vi "Dashboard Main.vi"() -> ()   [LabVIEW 2016]
uses:
  <vilib>/Utility/miscctls.llb/LVRowAndColumnTypeDef.ctl
  <vilib>/event_ctls.llb/eventvkey.ctl
  <vilib>/Rock Robotics/Network Tables/NT Read Numeric Array.vi
  <vilib>/Rock Robotics/WPI/Dashboard/WPI_DashboardLogging Global.vi
panel:
  in  "Camera Settings Right":T1={"Frame Rate"=30, "Compression"=30, "Size"=1, "DB Camera Config"=FALSE} {"Frame Rate" scale=1.0..30.0; "Compression" scale=100.0..-1.0; "Size" items=["640x480", "320x240", "160x120"]}
  in  "Camera Name Right":string(combo)="No Camera Selection"
  out "Camera Info":cluster{"Mbps LED":bool, "Mbps":dbl, "fps":dbl} {"fps" format="%#.1g"; "Mbps" format="%#.1g"}
  in  "Camera Settings":T1={"Frame Rate"=30, "Compression"=30, "Size"=1, "DB Camera Config"=FALSE} {"Frame Rate" scale=1.0..30.0; "Compression" scale=100.0..-1.0; "Size" items=["640x480", "320x240", "160x120"]}
  in  "TCP":refnum<k5>
  in  "Rec Mode":enum32{"Stop", "Record", "Playback"}(radio)
  out "Robot IP":string
  out "Image Message":string="Timeout in Camera Communications"
  in  "Dashboard Tab":T2(tab)
  in  "Select Auto":string(combo)="Select Autonomous ..."
  out "NT Connection":bool
  out "MotorChart R":cluster{"Numeric":dbl, "Numeric":dbl}(graph)
  out "MotorChart L":cluster{"Numeric":dbl, "Numeric":dbl}(graph)
  out "MotorSliders R":cluster{"MotorSlide1":dbl, "MotorSlide2":dbl} {"MotorSlide2" scale=-1.0..1.0 scale format="%#_2e"; "MotorSlide1" scale=-1.0..1.0 scale format="%#_2e"}
  out "MotorSliders L":cluster{"MotorSlide1":dbl, "MotorSlide2":dbl} {"MotorSlide2" scale=-1.0..1.0 scale format="%#_2e"; "MotorSlide1" scale=-1.0..1.0 scale format="%#_2e"}
  out "Gyro":dbl(knob) scale=0.0..360.0
  out "JS1 Z":dbl(slide) scale=-1.0..1.0 scale format="%#_2e"
  out "JS1 Graph":cluster{"X":dbl, "Y":dbl}[](graph)
  out "JS1 Buttons":T3
  out "JS2 Z":dbl(slide) scale=-1.0..1.0 scale format="%#_2e"
  out "JS2 Graph":cluster{"X":dbl, "Y":dbl}[](graph)
  out "JS2 Buttons":T3
  out "Mode":T4(ring)=enum."Auto Disabled"
  out "Camera Image Right":T5(plugin-control)
  in  "DB/String 9":string
  in  "DB/String 8":string
  in  "DB/String 7":string
  in  "DB/String 6":string
  in  "DB/String 5":string
  in  "DB/String 4":string
  in  "DB/String 3":string
  in  "DB/String 2":string
  in  "DB/String 1":string
  in  "DB/String 0":string
  in  "DB/Slider 0":dbl(slide) scale=0.0..5.0
  in  "DB/Slider 1":dbl(slide) scale=0.0..5.0
  in  "DB/Slider 2":dbl(slide) scale=0.0..5.0
  in  "DB/Slider 3":dbl(slide) scale=0.0..5.0
  out "DB/LED 3":bool
  out "DB/LED 2":bool
  out "DB/LED 1":bool
  out "DB/LED 0":bool
  in  "TimedDrive":bool
  in  "DriveTowardTower":bool caption="Tower Drive"
  in  "ReleaseGear":bool
  in  "GrabGear":bool
  in  "Test Slider":dbl(slide) scale=0.0..100.0 scale format="%#_3g"
  in  "On/Off":bool caption="Solenoid"
  in  "Test Name":u16(ring) items=["Select the test to run..."]
  in  "Test Tree":string(tree)
  in  "Motor":cluster{"Value":dbl, "Enable":bool} {"Value" scale=-1.0..1.0 scale format="%#_3g"}
  out "Progress":T6 {"Test Progress" scale=0.0..100.0}
  in  "Rev/Fwd":cluster{"Forward":bool, "Reverse":bool}
  in  "Test Ring":u16(ring) items=["Monochrome", "Color"]
  out "Cmd Status":string
  in  "Execute Command":bool
  in  "Command Params":string[][](table)
  in  "Command Selection":i32(listbox)
  in  "CheckList":i32(listbox)
  in  "Tree":string(tree)
  out "Camera Image":T5(plugin-control)
  out "Background":bool
  in  "Camera Name":string(combo)="No Camera Selection"
  # "HW"
  # "HW"
  # "Joysticks"
  # "Drive Motors"
  # "Front"
  # "Right"
  # "Left"
  # "Back"
  # "This tab is a great place for autonomous settings and robot-specific values.\nPlace controls and indicators inside this tab and match name to\nDashboard Variables on robot. You can also delete this comment."
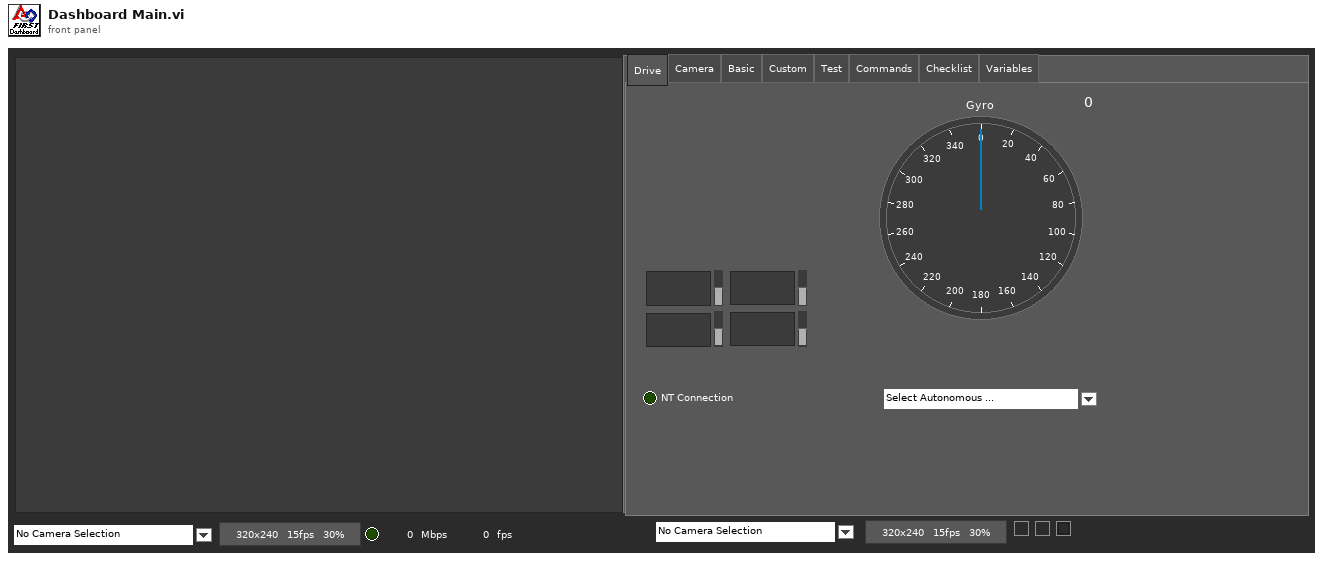
[diagram p1: front panel]
types:
  T1 = cluster{"Frame Rate":i32, "Compression":i32, "Size":u16, "DB Camera Config":bool}
  T2 = enum32{"Drive", "Camera", "Basic", "Custom", "Test", "Commands", "Checklist", "Variables"}
  T3 = cluster{bool, bool, bool, bool, bool, bool, bool, bool, bool, bool, bool, bool}
  T4 = enum8{"Tele-Op Disabled", "Tele-Op Enabled", "Auto Disabled", "Auto Enabled", "Test Disabled", "Test Enabled", "Disconnected", "No Code", "E-Stop"}
  T5 = typedef "IMAQ Image.ctl" = refnum<image>
  T6 = cluster{"Test Progress":u8, "Test Progress Text":string}
  T7 = typedef "Image Type" = u32
  T8 = cluster{"IDs":cluster{"RPC field ID":u16, "Unique ID":u16}, "String":string}
  T9 = enum32{"Drive", "Basic", "Custom", "Test", "Checklist", "Variables"}
  T10 = cluster{"Error Strings":string, "Disable Counts":cluster{u16, u16}, "Rail Faults":cluster{u16, u16, u16}, "Robot IP":string, "DB Mode":u8, "Event Info":cluster{"Name":string, "Type":u8, "Number":u16, "Replay":u8}}
  T11 = cluster{"Storage":cluster{"Disk Free":u64, "RAM Block":u32, "RAM free":u32}, "CPU Utilization":cluster{"CPU % ISR":sgl, "CPU % Time Crit":sgl, "CPU % Timed Str":sgl, "CPU % High":sgl, "CPU % Above":sgl, "CPU % Normal":sgl, "CPU % Low":sgl}, "CAN":cluster{"% Bus Utilization":sgl, "Bus Off Cnt":u32, "TX_FIFO Full Cnt":u32, "Receive Error Cnt":u8, "Transmit Error Cnt":u8}, "HID":cluster{"HID Outputs":u32, "Rumble Low":u16, "Rumble High":u16}[]}
  T12 = cluster{"Status bits":cluster{"Test Mode":bool, "Autonomous":bool, "Enabled":bool, "Code Start":bool, "Brownout":bool, "Reserved 2":bool, "Reserved 3":bool, "E-Stop":bool}, "Code Trace":cluster{"Disabled":bool, "TeleOp":bool, "Auto":bool, "Test":bool}, "Controller Type":enum16{"unknown", "cRIO", "roboRio"}, "Code?":enum16{"unknown", "noCode", "code"}, "Battery V":dbl}
  T13 = cluster{"Control Bits":cluster{"TestMode":bool, "Autonomous":bool, "Enabled":bool, "FMS Present":bool, bool, bool, bool, "E-Stop":bool}, "Team Station ":u8, "Countdown":sgl, "Joystick Values":cluster{"Axes":dbl[], "Buttons":bool[], "POVs":i16[]}[]}
  T14 = cluster{"Axes":dbl[], "Buttons":bool[], "POVs":i16[]}[]
  T15 = cluster{"Axes":dbl[], "Buttons":bool[], "POVs":i16[]}
  T16 = cluster{"Buttons[0]":bool, "Buttons[1]":bool, "Buttons[2]":bool, "Buttons[3]":bool, "Buttons[4]":bool, "Buttons[5]":bool, "Buttons[6]":bool, "Buttons[7]":bool, "Buttons[8]":bool, "Buttons[9]":bool, "Buttons[10]":bool, "Buttons[11]":bool}
  T17 = cluster{"Camera Image":refnum<vi>, "Dashboard Tab":refnum<vi>, "Background":refnum<vi>, "Rec Mode":refnum<vi>, "Test Slider":refnum<vi>, "On/Off ":refnum<vi>, "Test Ring":refnum<vi>, "Rev/Fwd":refnum<vi>, "Test Name":refnum<vi>, "Motor":refnum<vi>, "Progress":refnum<vi>, "CheckList":refnum<vi>, "Tree":refnum<vi>, "Test Tree":refnum<vi>, "Command Params":refnum<vi>, "Command Selection":refnum<vi>, "Execute Command":refnum<vi>, "Cmd Status":refnum<vi>, "Camera Settings":refnum<vi>, "Camera Name":refnum<vi>, "Camera Info":refnum<vi>, "Camera Settings Right":refnum<vi>, "Camera Name Right":refnum<vi>, "Camera Image Right":refnum<vi>}
  T18 = cluster{"Operation":enum16{"Update", "Clear"}, "Color Box":u32}[]
  T19 = typedef "eventvkey.ctl" = enum16{"ASCII", "Enter", "Return", "Shift", "Ctrl", "Alt", "Cmd", "Opt", "Caps", "NumLock", "Clear", "Break", "Up", "Down", "Left", "Right", "Insert", "Delete", "Home", "End", "PageUp", "PageDown", "Escape", "Help", "Pause", "ScrollLock", "F1", "F2", "F3", "F4", "F5", "F6", "F7", "F8", "F9", "F10", "F11", "F12", "F13", "F14", "F15", "F16", "F17", "F18", "F19", "F20", "F21", "F22", "F23", "F24", "Play", "VolumeUp", "VolumeDown", "Mute", "Two Byte Char"}
  T20 = cluster{"Image Size":bool, "Image Type":bool, "Pixel Value":bool, "ROI Information":bool, "Zoom Factor":bool}
  T21 = cluster{"Operation":enum16{"Update", "Clear"}, "Color Box":u32}
  T22 = typedef "LVRowAndColumnTypeDef.ctl" = cluster{"Row":i32, "Column":i32}
  T23 = cluster{"Shift":bool, "Ctrl":bool, "Alt":bool, "Cmd":bool, "Opt":bool}
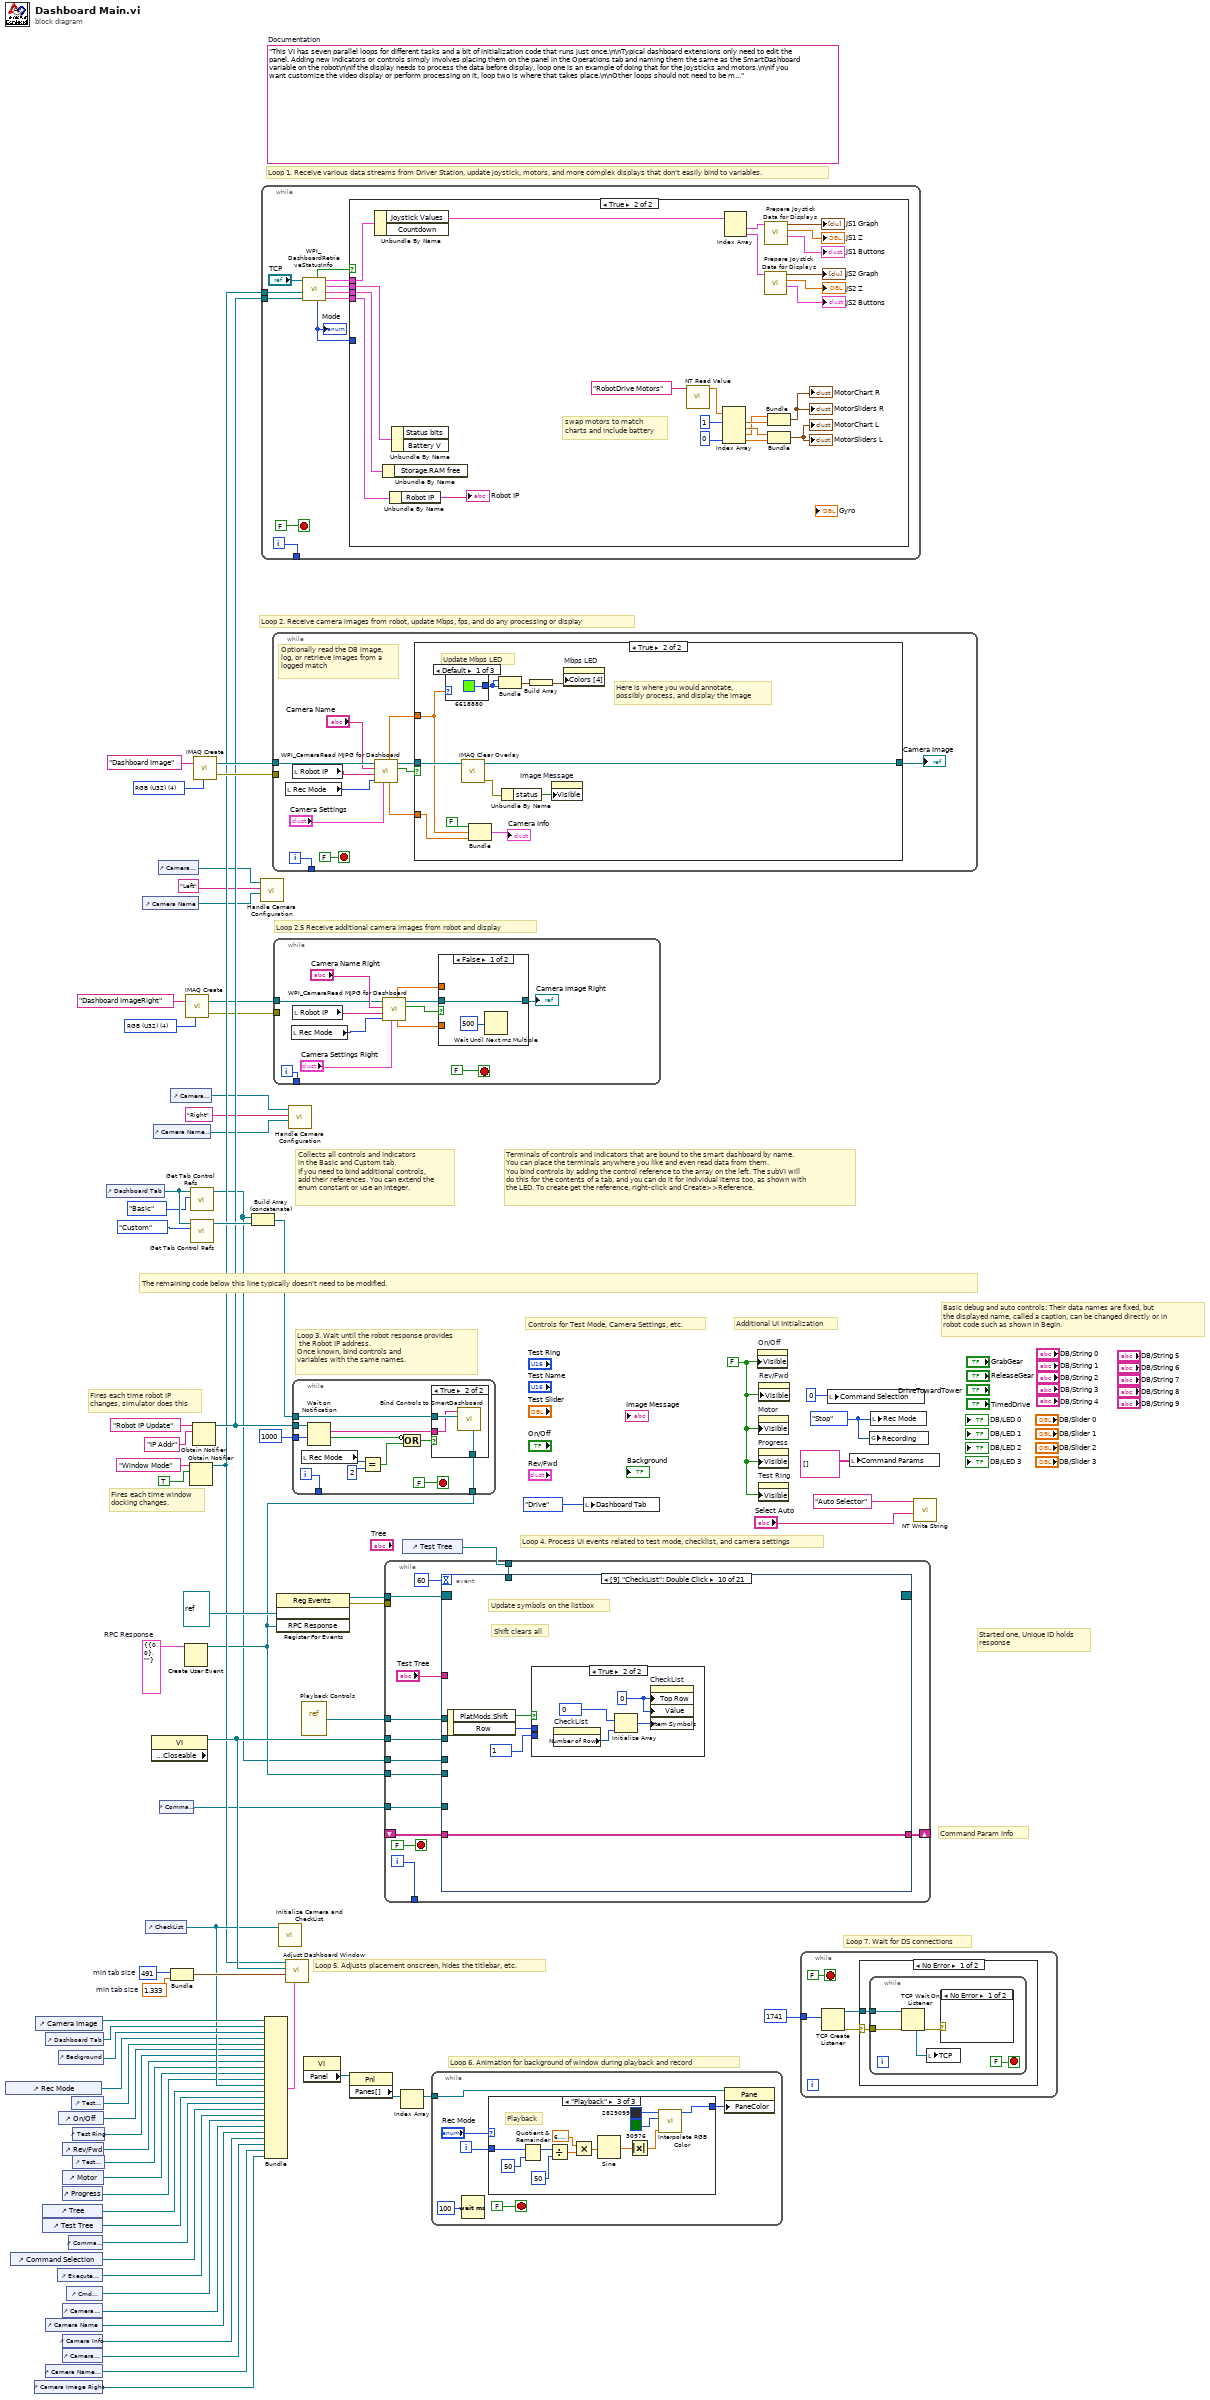
[diagram p0: block diagram]
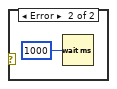
[diagram p3: hidden frame]
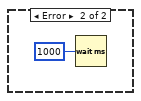
[diagram p4: hidden frame]
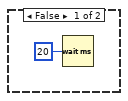
[diagram p5: hidden frame]
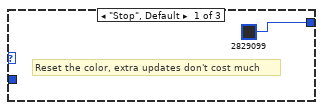
[diagram p6: hidden frame]
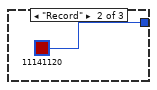
[diagram p7: hidden frame]
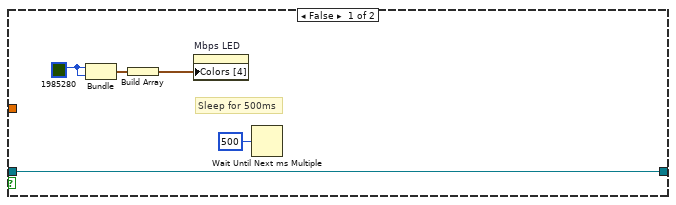
[diagram p9: hidden frame]
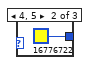
[diagram p10: hidden frame]
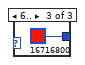
[diagram p11: hidden frame]
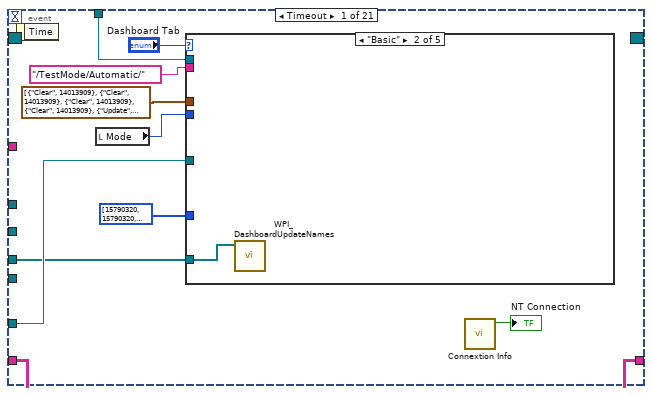
[diagram p12: hidden frame]
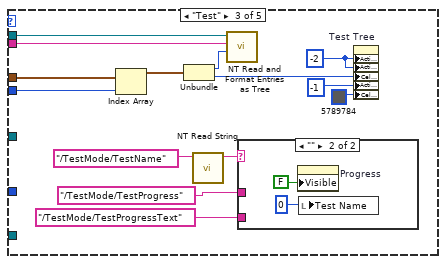
[diagram p14: hidden frame]
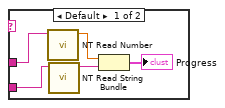
[diagram p15: hidden frame]
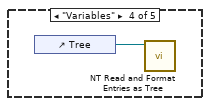
[diagram p16: hidden frame]
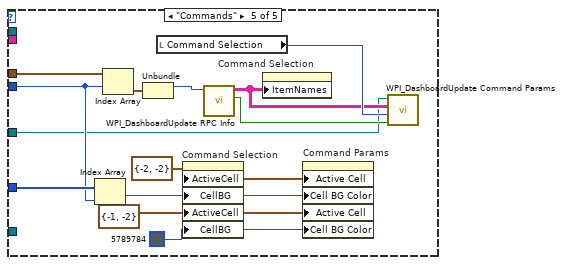
[diagram p17: hidden frame]
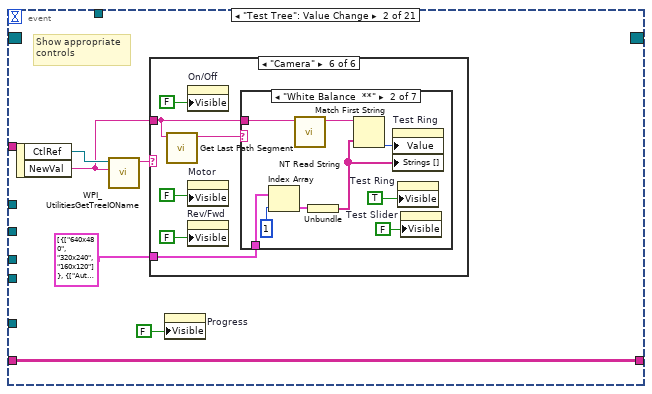
[diagram p18: hidden frame]
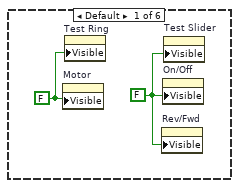
[diagram p19: hidden frame]
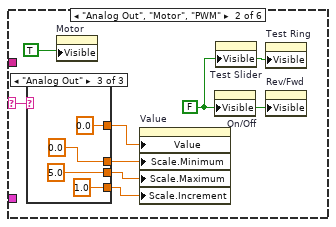
[diagram p20: hidden frame]
diagram:
  w10 = T7 4 items=["Grayscale (U8)", "Grayscale (I16)", "Grayscale (SGL)", "Complex (CSG)", "RGB (U32)", "HSL (U32)", "RGB (U64)"] ("Image Type")
  w26 = T8 {"IDs"={"RPC field ID"=0, "Unique ID"=0}, "String"=""}  # RPC Response
  w51 = 491  # min tab size
  w50 = 1.333  # min tab size
  w58 = enum32{"Stop", "Record", "Playback"}."Stop" ("Rec Mode")
  w33 = FALSE ("Visible")
  (unwired) "This VI has seven parallel loops for different tasks and a bit of initialization code that runs just once.\n\nTypical dashboard extensions only need to edit the panel. Adding new indicators or controls simply involves placing them on the panel in the Operations tab and naming them the same as the SmartDashboard variable on the robot\n\nIf the display needs to process the data before display, loop one is an example of doing that for the joysticks and motors.\n\nIf you want customize the video display or perform processing on it, loop two is where that takes place.\n\nOther loops should not need to be modified. They are pretty standard, and document the task they perform."  # Documentation
  w75 = T7 4 items=["Grayscale (U8)", "Grayscale (I16)", "Grayscale (SGL)", "Complex (CSG)", "RGB (U32)", "HSL (U32)", "RGB (U64)"] ("Image Type")
  # "Loop 2.5 Receive additional camera images from robot and display"
  # "Command Param Info"
  # "Started one, Unique ID holds\nresponse"
  # "Loop 7. Wait for DS connections"
  # "Basic debug and auto controls: Their data names are fixed, but\nthe displayed name, called a caption, can be changed directly or in\nrobot code such as shown in Begin."
  # "Controls for Test Mode, Camera Settings, etc."
  # "Additional UI Initialization"
  # "Loop 6. Animation for background of window during playback and record"
  # "Fires each time robot IP\nchanges, simulator does this"
  # "Fires each time window\ndocking changes."
  # "Collects all controls and indicators\nin the Basic and Custom tab.\nIf you need to bind additional controls,\nadd their references. You can extend the\nenum constant or use an integer."
  # "The remaining code below this line typically doesn't need to be modified."
  # "Loop 4. Process UI events related to test mode, checklist, and camera settings"
  # "Terminals of controls and indicators that are bound to the smart dashboard by name.\nYou can place the terminals anywhere you like and even read data from them.\nYou bind controls by adding the control reference to the array on the left. The subVI will\ndo this for the contents of a tab, and you can do it for individual items too, as shown with\nthe LED. To create get the reference, right-click and Create>>Reference."
  # "Loop 3. Wait until the robot response provides\n the Robot IP address.\nOnce known, bind controls and\nvariables with the same names."
  # "Loop 5. Adjusts placement onscreen, hides the titlebar, etc."
  # "Loop 1. Receive various data streams from Driver Station, update joystick, motors, and more complex displays that don't easily bind to variables."
  # "Loop 2. Receive camera images from robot, update Mbps, fps, and do any processing or display"
  n1 = control-ref of="Rec Mode"() -> (w39:refnum<vi>)
  n2 = control-ref of="Command Selection"() -> (w25:refnum<vi>)
  n3 = control-ref of="Camera Image Right"() -> (w1:refnum<vi>)
  n4 = control-ref of="Camera Image"() -> (w53:refnum<vi>)
  n5 = control-ref of="Tree"() -> (w43:refnum<vi>)
  n6 = control-ref of="Test Tree"() -> (w42:refnum<vi>)
  n7 = control-ref of="Dashboard Tab"() -> (w52:refnum<vi>)
  n8 = control-ref of="Camera Name"() -> (w16:refnum<vi>)
  n9 = control-ref of="Camera Name Right"() -> (w2:refnum<vi>)
  n10 = control-ref of="Execute Command"() -> (w27:refnum<vi>)
  n11 = control-ref of="Background"() -> (w48:refnum<vi>)
  n12 = control-ref of="On/Off"() -> (w37:refnum<vi>)
  n13 = control-ref of="Progress"() -> (w34:refnum<vi>)
  n14 = control-ref of="Camera Settings"() -> (w17:refnum<vi>)
  n15 = control-ref of="Camera Info"() -> (w15:refnum<vi>)
  n16 = control-ref of="Camera Settings Right"() -> (w3:refnum<vi>)
  n17 = control-ref of="Rev/Fwd"() -> (w35:refnum<vi>)
  n18 = control-ref of="Motor"() -> (w40:refnum<vi>)
  n19 = control-ref of="Cmd Status"() -> (w21:refnum<vi>)
  n20 = control-ref of="Command Params"() -> (w28:refnum<vi>)
  n21 = control-ref of="Test Slider"() -> (w38:refnum<vi>)
  n22 = control-ref of="Test Ring"() -> (w36:refnum<vi>)
  n23 = control-ref of="Test Name"() -> (w41:refnum<vi>)
  n24 = control-ref of="Dashboard Tab"() -> (w56:refnum<vi>)
  n25 = control-ref of="Camera Name"() -> (w18:refnum<vi>)
  n26 = control-ref of="CheckList"() -> (w44:refnum<vi>)
  n27 = property class="VI" props=["Front Panel.Closeable"]() -> (reference out=w57:refnum<vi>)  [unwired: 2 in, 2 out]
  n28 = control-ref of="Camera Name Right"() -> (w6:refnum<vi>)
  n29 = control-ref of="Camera Settings"() -> (w19:refnum<vi>)
  n30 = control-ref of="Command Params"() -> (w20:refnum<vi>)
  n31 = control-ref of="Camera Settings Right"() -> (w7:refnum<vi>)
  n32 = Bundle("min tab size"=w51, "min tab size"=w50) -> (w49:cluster{"min tab size":i32, "min tab size":dbl})  [unwired: 1 in]
  n33 = Create User Event(user event datatype=w26) -> (user event=w22:refnum<user-event>)  [unwired: 1 in, 1 out]
  n34 = call "IMAQ Create"("Image Name"="Dashboard ImageRight", "Image Type"=w10) -> ("New Image"=w9:T5, "error out"=w8:errorcluster)  [unwired: 2 in, 1 out]
  n35 = Obtain Notifier(name (unnamed)="Window Mode", notification data type=TRUE) -> (notifier out=w31:refnum<notifier>)  [unwired: 2 in, 2 out]
  n36 = call <vilib>:"Get Tab Control Refs.vi"("Page Index"=T9."Basic" ("Dashboard Tab"), "TabControl in"=w56) -> ("ControlsOnPage"=w14:refnum<vi>[])  [unwired: 9 in]
  n37 = call <vilib>:"Get Tab Control Refs.vi"("Page Index"=T9."Custom" ("Dashboard Tab"), "TabControl in"=w56) -> ("ControlsOnPage"=w55:refnum<vi>[])  [unwired: 9 in]
  n38 = Obtain Notifier(name (unnamed)="Robot IP Update", notification data type="IP Addr" ("name (unnamed)")) -> (notifier out=w32:refnum<notifier>)  [unwired: 2 in, 2 out]
  n39 = call "IMAQ Create"("Image Name"="Dashboard Image", "Image Type"=w75) -> ("New Image"=w73:T5, "error out"=w72:errorcluster)  [unwired: 2 in, 1 out]
  n40 = Build Array (concatenate)(w14, w55) -> (w54:refnum<vi>[])
  n41 = call "Handle Camera Configuration.vi"("CameraNameRef"=w18, "Camera File Name"="Left", "ClusterRef"=w19) -> ()  [unwired: 9 in]
  n42 = while {
    tunnel: [w85] -> _
    tunnel: w32 -> [w79]
    tunnel: w31 -> [w76]
    i -> [w85]
    stop <- FALSE stop-if-true
    n43 = call <vilib>:"WPI_DashboardRetrieveStatusInfo.vi"("Binding Refnum"=w79, "Window Mode Notifier"=w76, "TCP Cnx"="TCP") -> ("Power and Errors"=w80:T10, "Robot Metrics"=w83:T11, "Status Info"=w84:T12, "Control Info"=w81:T13, "Robot Mode"=w78:T4, "Process?"=w82:bool)  [unwired: 3 in]
    "Mode" <- w78
    n44 = case shown="True" w82 {
      tunnel: w84 -> [_ w111]
      tunnel: w83 -> [_ w110]
      tunnel: w81 -> [_ w109]
      tunnel: w80 -> [_ w108]
      tunnel: w78 -> [_ _]
      frame False {
        n45 = Wait (ms)(milliseconds to wait=u32 20) -> ()  [unwired: 1 out]
      }
      frame True {
        # "swap motors to match\ncharts and include battery"
        n46 = Unbundle By Name(w109) -> ("Joystick Values"=w99:T14)  [unwired: 1 out]
        n47 = Unbundle By Name(w110) -> ()  [unwired: 1 out]
        n48 = Unbundle By Name(w108) -> ("Robot IP"=→"Robot IP":string)
        n49 = Unbundle By Name(w111) -> ()  [unwired: 2 out]
        n50 = call-poly <vilib>:"NT Read Value.vi"("Name"="RobotDrive Motors") -> ("Numeric Array"=w89:dbl[])  [unwired: 9 in, 1 out]
        n51 = Index Array(array=w89, index #1=1, index #4=0) -> (element #1=w103:dbl, element #2=w104:dbl, element #3=w102:dbl, element #4=w107:dbl)  [unwired: 2 in]
        n52 = Index Array(array=w99) -> (element #1=w98:T15, element #2=w94:T15)  [unwired: 2 in]
        n53 = call "Prepare Joystick Data for Displays.vi"("Joystick Values"=w94) -> ("Buttons"=→"JS2 Buttons":T16, "Z Axis"=→"JS2 Z":dbl, "Cartesian Data"=→"JS2 Graph":cluster{"X axis":dbl, "X axis":dbl}[])  [unwired: 8 in]
        n54 = call "Prepare Joystick Data for Displays.vi"("Joystick Values"=w98) -> ("Buttons"=→"JS1 Buttons":T16, "Z Axis"=→"JS1 Z":dbl, "Cartesian Data"=→"JS1 Graph":cluster{"X axis":dbl, "X axis":dbl}[])  [unwired: 8 in]
        n55 = Bundle("Numeric"=w102, "Numeric"=w103) -> (→"MotorChart R" →"MotorSliders R":cluster{"Numeric":dbl, "Numeric":dbl})  [unwired: 1 in]
        n56 = Bundle("Numeric"=w104, "Numeric"=w107) -> (→"MotorChart L" →"MotorSliders L":cluster{"Numeric":dbl, "Numeric":dbl})  [unwired: 1 in]
      }
    }
  }
  n57 = Bundle("Camera Image"=w53, "Dashboard Tab"=w52, "Background"=w48, "Rec Mode"=w39, "Test Slider"=w38, "On/Off"=w37, "Test Ring"=w36, "Rev/Fwd"=w35, "Test Name"=w41, "Motor"=w40, "Progress"=w34, "CheckList"=w44, "Tree"=w43, "Test Tree"=w42, "Command Params"=w28, "Command Selection"=w25, "Execute Command"=w27, "Cmd Status"=w21, "Camera Settings"=w17, "Camera Name"=w16, "Camera Info"=w15, "Camera Settings Right"=w3, "Camera Name Right"=w2, "Camera Image Right"=w1) -> (w45:T17)  [unwired: 1 in]
  n58 = while {
    tunnel: w73 -> [w121]
    tunnel: w72 -> [_]
    tunnel: [w122] -> _
    i -> [w122]
    stop <- FALSE stop-if-true
    # "Optionally read the DB image,\nlog, or retrieve images from a\nlogged match"
    n59 = local read "Rec Mode"() -> (w117:enum32{"Stop", "Record", "Playback"})
    n60 = local read "Robot IP"() -> (w116:string)
    n61 = call <vilib>:"WPI_CameraRead MJPG for Dashboard.vi"("Camera Settings"="Camera Settings", "Rec Mode"=w117, "Robot IP"=w116, "Camera Name"="Camera Name", "Refnum in"=w121) -> ("Active"=w119:bool, "Refnum out"=w120:T5, "FPS"=w118:dbl, "Bandwidth (Mbps)"=w115:dbl)  [unwired: 3 in]
    n62 = case shown="True" w119 {
      tunnel: w120 -> [w124 w135]
      tunnel: w115 -> [_ w132]
      tunnel: w118 -> [_ w133]
      tunnel: [w124 w129] -> w112
      frame False {
        w126 = u32 1985280 ("Color Box")
        # "Sleep for 500ms"
        n63 = Bundle("Color Box"=w126, "Color Box"=w126) -> (w127:cluster{"Color Box":u32, "Color Box":u32})  [unwired: 1 out]
        n64 = Build Array(w127) -> (w125:cluster{"Color Box":u32, "Color Box":u32}[])
        n65 = property on="Mbps LED" class="Bool (strict)"("Colors [4]"=w125) -> ()  [unwired: 2 in, 2 out]
        n66 = Wait Until Next ms Multiple(millisecond multiple=u32 500) -> ()  [unwired: 1 out]
      }
      frame True {
        # "Here is where you would annotate,\npossibly process, and display the image"
        # "Update Mbps LED"
        n67 = case shown="Default" w132 {
          tunnel: [u32 6618880 ("Color Box") u32 16776722 ("Color Box") u32 16716800 ("Color Box")] -> w136
          frame Default {
          }
          frame 4, 5 {
          }
          frame 6.. {
          }
        }
        n68 = call "IMAQ Clear Overlay"("Image"=w135) -> ("error out"=w138:errorcluster, "Image Out"=w129:T5)  [unwired: 2 in, 7 out]
        n69 = Bundle(FALSE, "Bandwidth (Mbps)"=w132, "FPS"=w133) -> (→"Camera Info":cluster{bool, "Bandwidth (Mbps)":dbl, "FPS":dbl})  [unwired: 1 in]
        n70 = Bundle("Color Box"=w136, "Color Box"=w136) -> (w137:cluster{"Color Box":u32, "Color Box":u32})  [unwired: 1 out]
        n71 = Unbundle By Name(w138) -> ("status"=w139:bool)
        n72 = Build Array(w137) -> (w134:cluster{"Color Box":u32, "Color Box":u32}[])
        n73 = property on="Image Message" class="Str"("Visible"=w139) -> ()  [unwired: 2 in, 2 out]
        n74 = property on="Mbps LED" class="Bool (strict)"("Colors [4]"=w134) -> ()  [unwired: 2 in, 2 out]
      }
    }
    "Camera Image" <- w112
  }
  n75 = while {
    tunnel: w9 -> [w153]
    tunnel: w8 -> [_]
    tunnel: [w147] -> _
    i -> [w147]
    stop <- FALSE stop-if-true
    n76 = local read "Rec Mode"() -> (w151:enum32{"Stop", "Record", "Playback"})
    n77 = local read "Robot IP"() -> (w152:string)
    n78 = call <vilib>:"WPI_CameraRead MJPG for Dashboard.vi"("Camera Settings"="Camera Settings Right", "Rec Mode"=w151, "Robot IP"=w152, "Camera Name"="Camera Name Right", "Refnum in"=w153) -> ("Active"=w146:bool, "Refnum out"=w149:T5, "FPS"=w144:dbl, "Bandwidth (Mbps)"=w145:dbl)  [unwired: 3 in]
    n79 = case shown="False" w146 {
      tunnel: w149 -> [w155 w157]
      tunnel: w145 -> [_ _]
      tunnel: w144 -> [_ _]
      tunnel: [w155 w157] -> w143
      frame False {
        n80 = Wait Until Next ms Multiple(millisecond multiple=u32 500) -> ()  [unwired: 1 out]
      }
      frame True {
      }
    }
    "Camera Image Right" <- w143
  }
  n81 = register-events(refnum<vi> refnum, w22) -> (reference out=w62:refnum<event-registration>, error out=w61:errorcluster)  [unwired: 2 in]
  n82 = call "Initialize Camera and CheckList.vi"("ListBox in"=w44) -> ()  [unwired: 11 in]
  n83 = call "Adjust Dashboard Window.vi"("Sizing Refnums"=w45, "Size Constraints"=w49, "VI"=w57, "WIn Mode"=w31) -> ()  [unwired: 8 in]
  n84 = call "Handle Camera Configuration.vi"("CameraNameRef"=w6, "Camera File Name"="Right", "ClusterRef"=w7) -> ()  [unwired: 9 in]
  n85 = while {
    tunnel: w54 -> [w169]
    tunnel: w32 -> [w167]
    tunnel: [w165] -> _
    tunnel: u32 1000 ("milliseconds to wait") -> [w164]
    tunnel: w22 -> [w158]
    i -> [w165]
    stop <- FALSE stop-if-true
    n86 = local read "Rec Mode"() -> (w160:enum32{"Stop", "Record", "Playback"})
    n87 = Wait on Notification(notifier=w167, timeout in ms (-1)=w164) -> (notification=w166:string, timed out?=w162:bool)  [unwired: 2 in, 2 out]
    n88 = Equal?(x=w160, y=u16 2 ("Rec Mode")) -> (x = y?=w161:bool)
    n89 = Compound Arithmetic op=OR(invert w162, w161) -> (w163:bool)
    n90 = case shown="True" w163 {
      tunnel: w169 -> [_ w172]
      tunnel: w166 -> [_ w171]
      tunnel: w158 -> [_ w170]
      frame False {
      }
      frame True {
        n91 = call <vilib>:"Bind Controls to SmartDashboard.vi"("RPC ref"=w170, "Bound Control Refs"=w172, "Server IP Address"=w171) -> ()  [unwired: 9 in]
      }
    }
  }
  n92 = vi-ref "Playback Controls.vi"() -> (w63:refnum<vi>)
  n93 = property class="VI"() -> ("Panel"=w65:refnum<vi>)  [unwired: 2 in, 2 out]
  n94 = property class="Pnl"(reference=w65) -> ("Panes[]"=w66:refnum<vi>[])  [unwired: 1 in, 2 out]
  n95 = Index Array(array=w66) -> (element=w64:refnum<vi>)  [unwired: 1 in]
  n96 = control-ref of="Test Tree"() -> (w67:refnum<vi>)
  n97 = while {
    tunnel: [w182] -> _
    tunnel: w67 -> [w181]
    tunnel: w63 -> [w180]
    tunnel: w62 -> [w179]
    tunnel: w61 -> [_]
    tunnel: w57 -> [w178]
    tunnel: w22 -> [w177]
    tunnel: w20 -> [w176]
    shift-right: [w175] -> _
    shift-left: _ -> [w174]
    tunnel: w14 -> [w173]
    i -> [w182]
    stop <- FALSE stop-if-true
    n98 = event shown="[9] \"CheckList\": Double Click" {
      selector: w179 -> [_ _ _ _ _ _ _ _ _ _ _ _ _ _ _ _ _ _ _ _ _]
      dyn-events: [_ _ _ _ _ _ _ _ _ _ _ _ _ _ _ _ w438 _ _ _ _] -> _
      timeout: u32 60 ("milliseconds to wait") -> [_ _ _ _ _ _ _ _ _ _ _ _ _ _ _ _ _ _ _ _ _]
      tunnel: w181 -> [w194 _ _ _ _ _ _ _ _ _ _ _ _ _ _ _ _ _ _ _ _]
      tunnel: "Test Tree" -> [_ _ _ _ _ _ _ _ _ _ _ w405 w413 w415 w419 w427 _ _ _ _ _]
      tunnel: w180 -> [_ _ _ _ _ _ _ _ _ _ _ _ _ _ _ _ w440 _ w458 _ _]
      tunnel: w178 -> [_ _ _ _ _ _ _ _ _ _ _ _ _ _ _ _ w436 _ _ _ _]
      tunnel: w177 -> [_ _ _ _ _ _ _ _ _ _ _ _ _ _ _ _ w432 _ _ _ _]
      tunnel: w176 -> [w189 _ _ _ _ _ w356 _ _ _ _ _ _ _ _ _ _ _ _ _ _]
      tunnel: [w188 w233 w335 w340 w349 w353 w354 w363 w373 w380 w392 w404 w411 w414 w418 w426 w431 w453 w455 w459 w470] -> w175
      tunnel: w174 -> [w188 w233 w335 w340 w349 w353 w354 _ _ w380 w392 w404 w411 w414 w418 w426 w431 w453 w455 w459 w470]
      tunnel: w173 -> [w186 _ _ _ _ _ _ _ _ _ _ _ _ _ _ _ _ _ _ _ _]
      event Timeout {
        n99 = event-data() -> ()  [unwired: 1 in, 1 out]
        n100 = local read "Mode"() -> (w191:T4)
        n101 = case shown="\"Basic\"" "Dashboard Tab" {
          tunnel: w194 -> [_ _ w210 _ _]
          tunnel: "/TestMode/Automatic/" ("Name Pattern") -> [_ _ w209 _ _]
          tunnel: T18 [{"Operation"=enum."Clear", "Color Box"=14013909}, {"Operation"=enum."Clear", "Color Box"=14013909}, {"Operation"=enum."Clear", "Color Box"=14013909}, {"Operation"=enum."Clear", "Color Box"=14013909}, {"Operation"=enum."Update", "Color Box"=14013909}, {"Operation"=enum."Update", "Color Box"=16777215}, {"Operation"=enum."Clear", "Color Box"=14013909}, {"Operation"=enum."Clear", "Color Box"=14013909}, {"Operation"=enum."Clear", "Color Box"=14013909}] -> [_ _ w202 _ w226]
          tunnel: w191 -> [_ _ w201 _ w225]
          tunnel: u32[] [15790320, 15790320, 15790320, 15790320, 16777215, 16777215, 15790320, 15790320, 15790320] -> [_ _ _ _ w231]
          tunnel: w189 -> [_ _ _ _ w219]
          tunnel: w186 -> [_ w196 _ _ _]
          frame "Custom", Default {
          }
          frame "Basic" {
            n102 = call <vilib>:"WPI_DashboardUpdateNames.vi"("Controls on Tab"=w196) -> ()  [unwired: 11 in]
          }
          frame "Test" {
            w208 = -2 ("Active Item:Row Number")
            n103 = Index Array(array=w202, index=w201) -> (element=w203:T21)
            n104 = Unbundle(w203) -> ("Operation"=w204:enum16{"Update", "Clear"}, "Color Box"=w205:u32)
            n105 = call <vilib>:"NT Read String.vi"("Name"="/TestMode/TestName") -> ("String"=w199:string)  [unwired: 9 in, 1 out]
            n106 = call <vilib>:"NT Read and Format Entries as Tree.vi"("Operation"=w204, "Name Pattern"=w209, "Tree Refnum"=w210) -> ()  [unwired: 7 in, 2 out]
            n107 = case shown="\"\"" w199 {
              tunnel: "/TestMode/TestProgress" ("Name") -> [w212 _]
              tunnel: "/TestMode/TestProgressText" ("Name") -> [w211 _]
              frame Default {
                n108 = call <vilib>:"NT Read Number.vi"("Name"=w212) -> ("Numeric"=w213:dbl)  [unwired: 9 in, 1 out]
                n109 = call <vilib>:"NT Read String.vi"("Name"=w211) -> ("String"=w214:string)  [unwired: 9 in, 1 out]
                n110 = Bundle("Numeric"=w213, "String"=w214) -> (→"Progress":cluster{"Numeric":dbl, "String":string})  [unwired: 1 in]
              }
              frame "" {
                n111 = property on="Progress" class="Clust (strict)"("Visible"=FALSE) -> ()  [unwired: 2 in, 2 out]
                n112 = local write "Test Name"(u16 0) -> ()
              }
            }
            n113 = property on="Test Tree" class="Tree (strict)"("Active Item Row Number"=w208, "ActiveColNum"=w208, "CellBG"=w205, "Active Item Row Number"=-1 ("Active Item:Row Number"), "CellBG"=u32 5789784 ("Color Box")) -> ()  [unwired: 2 in, 2 out]
          }
          frame "Variables" {
            n114 = control-ref of="Tree"() -> (w218:refnum<vi>)
            n115 = call <vilib>:"NT Read and Format Entries as Tree.vi"("Tree Refnum"=w218) -> ()  [unwired: 9 in, 2 out]
          }
          frame "Commands" {
            w227 = u32 5789784 ("Color Box")
            w228 = T22 {"Row"=-1, "Column"=-2} ("Active Cell:Active Cell")
            w230 = T22 {"Row"=-2, "Column"=-2} ("Active Cell:Active Cell")
            n116 = Index Array(array=w231, index=w225) -> (element=w229:u32)
            n117 = Index Array(array=w226, index=w225) -> (element=w224:T21)
            n118 = Unbundle(w224) -> ("Operation"=w223:enum16{"Update", "Clear"})  [unwired: 1 out]
            n119 = local read "Command Selection"() -> (w222:i32)
            n120 = property on="Command Selection" class="MCListbox (strict)"("ActiveCell"=w230, "CellBG"=w229, "ActiveCell"=w228, "CellBG"=w227) -> ()  [unwired: 2 in, 2 out]
            n121 = call <vilib>:"WPI_DashboardUpdate RPC Info.vi"("Operation"=w223) -> ("update"=w221:bool, "commands"=w220:string[][])  [unwired: 9 in]
            n122 = property on="Command Selection" class="MCListbox (strict)"("ItemNames"=w220) -> ()  [unwired: 2 in, 2 out]
            n123 = property on="Command Params" class="Tbl (strict)"("Active Cell"=w230, "Cell BG Color"=w229, "Active Cell"=w228, "Cell BG Color"=w227) -> ()  [unwired: 2 in, 2 out]
            n124 = call <vilib>:"WPI_DashboardUpdate Command Params.vi"("Update"=w221, "NewVal"=w222, "Commands"=w220, "Param Tbl"=w219) -> ()  [unwired: 7 in, 1 out]
          }
        }
        n125 = call <vilib>:"Connextion Info.vi"() -> ("Connected"=→"NT Connection":bool)  [unwired: 10 in, 1 out]
      }
      event "Test Tree": Value Change {
        # "Show appropriate\ncontrols"
        n126 = event-data() -> ("CtlRef"=w236:refnum<vi>, "NewVal"=w234:string)  [unwired: 1 in]
        n127 = call <vilib>:"WPI_UtilitiesGetTreeIOName.vi"("NewVal"=w234, "TreeControl in"=w236) -> ("I/O Name"=w237:string)  [unwired: 9 in]
        n128 = case shown="\"Camera\"" w237 {
          selector: w237 -> [_ w244 _ w266 w275 _]
          tunnel: w234 -> [_ _ w263 w265 _ w282]
          tunnel: cluster{string[]}[] [{["640x480", "320x240", "160x120"]}, {["Auto", "Fixed indoor", "Fixed outdoor 1", "Fixed outdoor 2", "Fixed fluorescent 1", "Fixed fluorescent 2", "Hold current"]}, {["Auto", "Flicker-free 50 Hz", "Flicker-free 60 Hz", "Hold current"]}, {["None", "Prioritize frame rate", "Prioritize image quality"]}, {["Monochrome", "Color"]}] -> [_ _ _ _ _ w281]
          frame Default {
            w239 = FALSE ("Visible")
            w238 = FALSE ("Visible")
            n129 = property on="Motor" class="Clust (strict)"("Visible"=w238) -> ()  [unwired: 2 in, 2 out]
            n130 = property on="Test Ring" class="Ring (strict)"("Visible"=w238) -> ()  [unwired: 2 in, 2 out]
            n131 = property on="Rev/Fwd" class="Clust (strict)"("Visible"=w239) -> ()  [unwired: 2 in, 2 out]
            n132 = property on="On/Off" class="Bool (strict)"("Visible"=w239) -> ()  [unwired: 2 in, 2 out]
            n133 = property on="Test Slider" class="Slide (strict)"("Visible"=w239) -> ()  [unwired: 2 in, 2 out]
          }
          frame "Analog Out", "Motor", "PWM" {
            w245 = FALSE ("Visible")
            n134 = case shown="\"Analog Out\"" w244 {
              tunnel: [1.0 ("Value") -1.0 ("Value") 0.0 ("Value")] -> w243
              tunnel: [255.0 ("Value") 1.0 ("Value") 5.0 ("Value")] -> w242
              tunnel: [128.0 ("Value") 0.0 ("Value") 0.0 ("Value")] -> w241
              tunnel: [64.0 ("Value") 0.5 ("Value") 1.0 ("Value")] -> w240
              frame "PWM" {
              }
              frame "Motor", Default {
              }
              frame "Analog Out" {
              }
            }
            n135 = property on="Motor" class="Clust (strict)"("Visible"=TRUE) -> ()  [unwired: 2 in, 2 out]
            n136 = property on="Value" class="Slide (strict)"("Value"=w241, "Scale.Minimum"=w243, "Scale.Maximum"=w242, "Scale.Increment"=w240) -> ()  [unwired: 2 in, 2 out]
            n137 = property on="On/Off" class="Bool (strict)"("Visible"=w245) -> ()  [unwired: 2 in, 2 out]
            n138 = property on="Test Slider" class="Slide (strict)"("Visible"=w245) -> ()  [unwired: 2 in, 2 out]
            n139 = property on="Test Ring" class="Ring (strict)"("Visible"=w245) -> ()  [unwired: 2 in, 2 out]
            n140 = property on="Rev/Fwd" class="Clust (strict)"("Visible"=w245) -> ()  [unwired: 2 in, 2 out]
          }
          frame "Servo" {
            w261 = FALSE ("Visible")
            n141 = call <vilib>:"NT Read Number.vi"("Name"=w263) -> ("Numeric"=w262:dbl)  [unwired: 9 in, 1 out]
            n142 = property on="Test Slider" class="Slide (strict)"("Visible"=TRUE, "Scale.Maximum"=170.0 ("Scale.Range:Maximum")) -> ()  [unwired: 2 in, 2 out]
            n143 = local write "Test Slider"(w262) -> ()
            n144 = property on="Motor" class="Clust (strict)"("Visible"=w261) -> ()  [unwired: 2 in, 2 out]
            n145 = property on="Rev/Fwd" class="Clust (strict)"("Visible"=w261) -> ()  [unwired: 2 in, 2 out]
            n146 = property on="On/Off" class="Bool (strict)"("Visible"=w261) -> ()  [unwired: 2 in, 2 out]
            n147 = property on="Test Ring" class="Ring (strict)"("Visible"=w261) -> ()  [unwired: 2 in, 2 out]
          }
          frame "Relay", "Solenoid" {
            w264 = FALSE ("Visible")
            n148 = property on="Motor" class="Clust (strict)"("Visible"=w264) -> ()  [unwired: 2 in, 2 out]
            n149 = property on="Test Slider" class="Slide (strict)"("Visible"=w264) -> ()  [unwired: 2 in, 2 out]
            n150 = Search and Replace String(input string=w265, search string="/Value  **", replace string="/Direction") -> (result string=w271:string)  [unwired: 5 in, 3 out]
            n151 = property on="Test Ring" class="Ring (strict)"("Visible"=w264) -> ()  [unwired: 2 in, 2 out]
            n152 = call <vilib>:"NT Read String.vi"("Name"=w271) -> ("String"=w269:string)  [unwired: 9 in, 1 out]
            n153 = Equal?(x="Both directions", y=w269) -> (x = y?=w267:bool)
            n154 = Not(x=w267) -> (.not. x?=w268:bool)
            n155 = property on="Rev/Fwd" class="Clust (strict)"("Visible"=w267) -> ()  [unwired: 2 in, 2 out]
            n156 = property on="On/Off" class="Bool (strict)"("Visible"=w268, "Caption.Text"=w266) -> ()  [unwired: 2 in, 2 out]
          }
          frame "Compressor", "Digital Out" {
            w274 = FALSE ("Visible")
            # "Get direction and finish"
            n157 = property on="Motor" class="Clust (strict)"("Visible"=w274) -> ()  [unwired: 2 in, 2 out]
            n158 = property on="Test Slider" class="Slide (strict)"("Visible"=w274) -> ()  [unwired: 2 in, 2 out]
            n159 = property on="Test Ring" class="Ring (strict)"("Visible"=w274) -> ()  [unwired: 2 in, 2 out]
            n160 = property on="On/Off" class="Bool (strict)"("Visible"=TRUE, "Caption.Text"=w275) -> ()  [unwired: 2 in, 2 out]
            n161 = property on="Rev/Fwd" class="Clust (strict)"("Visible"=FALSE) -> ()  [unwired: 2 in, 2 out]
          }
          frame "Camera" {
            n162 = call <vilib>:"Get Last Path Segment.vi"("String in"=w282) -> ("String out"=w283:string)  [unwired: 10 in]
            n163 = property on="On/Off" class="Bool (strict)"("Visible"=FALSE) -> ()  [unwired: 2 in, 2 out]
            n164 = property on="Motor" class="Clust (strict)"("Visible"=FALSE) -> ()  [unwired: 2 in, 2 out]
            n165 = property on="Rev/Fwd" class="Clust (strict)"("Visible"=FALSE) -> ()  [unwired: 2 in, 2 out]
            n166 = case shown="\"White Balance  **\"" w283 {
              tunnel: w282 -> [w289 w298 w307 w316 w325 _ w331]
              tunnel: w281 -> [w287 w295 w304 w313 w322 _ _]
              frame "Size  **" {
                n167 = Index Array(array=w287) -> (element=w286:cluster{string[]})  [unwired: 1 in]
                n168 = call <vilib>:"NT Read String.vi"("Name"=w289) -> ("String"=w288:string)  [unwired: 9 in, 1 out]
                n169 = Unbundle(w286) -> (w284:string[])
                n170 = Match First String(2:w284, 3:w288) -> (0:w285:i32)  [unwired: 1 out]
                n171 = property on="Test Ring" class="Ring (strict)"("Value"=w285, "Strings []"=w284) -> ()  [unwired: 2 in, 2 out]
                n172 = property on="Test Ring" class="Ring (strict)"("Visible"=TRUE) -> ()  [unwired: 2 in, 2 out]
                n173 = property on="Test Slider" class="Slide (strict)"("Visible"=FALSE) -> ()  [unwired: 2 in, 2 out]
              }
              frame "White Balance  **" {
                n174 = Index Array(array=w295, index=1) -> (element=w296:cluster{string[]})
                n175 = call <vilib>:"NT Read String.vi"("Name"=w298) -> ("String"=w297:string)  [unwired: 9 in, 1 out]
                n176 = Unbundle(w296) -> (w293:string[])
                n177 = Match First String(2:w293, 3:w297) -> (0:w292:i32)  [unwired: 1 out]
                n178 = property on="Test Ring" class="Ring (strict)"("Value"=w292, "Strings []"=w293) -> ()  [unwired: 2 in, 2 out]
                n179 = property on="Test Ring" class="Ring (strict)"("Visible"=TRUE) -> ()  [unwired: 2 in, 2 out]
                n180 = property on="Test Slider" class="Slide (strict)"("Visible"=FALSE) -> ()  [unwired: 2 in, 2 out]
              }
              frame "Exposure  **" {
                n181 = Index Array(array=w304, index=2) -> (element=w305:cluster{string[]})
                n182 = call <vilib>:"NT Read String.vi"("Name"=w307) -> ("String"=w306:string)  [unwired: 9 in, 1 out]
                n183 = Unbundle(w305) -> (w301:string[])
                n184 = Match First String(2:w301, 3:w306) -> (0:w302:i32)  [unwired: 1 out]
                n185 = property on="Test Ring" class="Ring (strict)"("Value"=w302, "Strings []"=w301) -> ()  [unwired: 2 in, 2 out]
                n186 = property on="Test Ring" class="Ring (strict)"("Visible"=TRUE) -> ()  [unwired: 2 in, 2 out]
                n187 = property on="Test Slider" class="Slide (strict)"("Visible"=FALSE) -> ()  [unwired: 2 in, 2 out]
              }
              frame "Exposure Priority  **" {
                n188 = Index Array(array=w313, index=3) -> (element=w314:cluster{string[]})
                n189 = call <vilib>:"NT Read String.vi"("Name"=w316) -> ("String"=w315:string)  [unwired: 9 in, 1 out]
                n190 = Unbundle(w314) -> (w310:string[])
                n191 = Match First String(2:w310, 3:w315) -> (0:w311:i32)  [unwired: 1 out]
                n192 = property on="Test Ring" class="Ring (strict)"("Value"=w311, "Strings []"=w310) -> ()  [unwired: 2 in, 2 out]
                n193 = property on="Test Ring" class="Ring (strict)"("Visible"=TRUE) -> ()  [unwired: 2 in, 2 out]
                n194 = property on="Test Slider" class="Slide (strict)"("Visible"=FALSE) -> ()  [unwired: 2 in, 2 out]
              }
              frame "Color Enable  **" {
                n195 = Index Array(array=w322, index=4) -> (element=w323:cluster{string[]})
                n196 = call <vilib>:"NT Read String.vi"("Name"=w325) -> ("String"=w324:string)  [unwired: 9 in, 1 out]
                n197 = Unbundle(w323) -> (w319:string[])
                n198 = Match First String(2:w319, 3:w324) -> (0:w320:i32)  [unwired: 1 out]
                n199 = property on="Test Ring" class="Ring (strict)"("Value"=w320, "Strings []"=w319) -> ()  [unwired: 2 in, 2 out]
                n200 = property on="Test Ring" class="Ring (strict)"("Visible"=TRUE) -> ()  [unwired: 2 in, 2 out]
                n201 = property on="Test Slider" class="Slide (strict)"("Visible"=FALSE) -> ()  [unwired: 2 in, 2 out]
              }
              frame Default {
                n202 = property on="Test Ring" class="Ring (strict)"("Visible"=FALSE) -> ()  [unwired: 2 in, 2 out]
                n203 = property on="Test Slider" class="Slide (strict)"("Visible"=FALSE) -> ()  [unwired: 2 in, 2 out]
              }
              frame "Brightness  **", "Color Level  **", "Compression  **", "FPS  **", "Sharpness  **" {
                n204 = call <vilib>:"NT Read Number.vi"("Name"=w331) -> ("Numeric"=w330:dbl)  [unwired: 9 in, 1 out]
                n205 = local write "Test Slider"(w330) -> ()
                n206 = property on="Test Slider" class="Slide (strict)"("Visible"=TRUE, "Scale.Maximum"=100.0 ("Scale.Range:Maximum")) -> ()  [unwired: 2 in, 2 out]
                n207 = property on="Test Ring" class="Ring (strict)"("Visible"=FALSE) -> ()  [unwired: 2 in, 2 out]
              }
            }
          }
        }
        n208 = property on="Progress" class="Clust (strict)"("Visible"=FALSE) -> ()  [unwired: 2 in, 2 out]
      }
      event "Test Name": Mouse Enter {
        # "Populate the ring with the list of tests"
        n209 = event-data() -> ()  [unwired: 1 in, 1 out]
        n210 = call <vilib>:"NT Read String Array.vi"("Name"="/TestMode/TestList") -> ("String Array"=w339:string[])  [unwired: 9 in, 1 out]
        n211 = Build Array (concatenate)("Select the test to run...", w339) -> (w338:string[])
        n212 = property on="Test Name" class="Ring (strict)"("Strings []"=w338) -> ()  [unwired: 2 in, 2 out]
      }
      event "Test Name": Value Change {
        w341 = FALSE ("Visible")
        # "Tell the robot the test name to run"
        n213 = event-data() -> ("NewVal"=w345:u16)  [unwired: 1 in]
        n214 = property on="Test Name" class="Ring (strict)"() -> ("Strings []"=w346:string[])  [unwired: 2 in, 2 out]
        n215 = local write "Progress"(T6 {"Test Progress"=0, "Test Progress Text"=""} ("Progress")) -> ()
        n216 = Index Array(array=w346, index=w345) -> (element=w344:string)
        n217 = call <vilib>:"NT Write String.vi"("String"=w344, "Name"="/TestMode/TestName") -> ()  [unwired: 9 in, 1 out]
        n218 = property on="Progress" class="Clust (strict)"("Visible"=TRUE) -> ()  [unwired: 2 in, 2 out]
        n219 = property on="Motor" class="Clust (strict)"("Visible"=w341) -> ()  [unwired: 2 in, 2 out]
        n220 = property on="Test Slider" class="Slide (strict)"("Visible"=w341) -> ()  [unwired: 2 in, 2 out]
        n221 = property on="On/Off" class="Bool (strict)"("Visible"=w341) -> ()  [unwired: 2 in, 2 out]
        n222 = property on="Rev/Fwd" class="Clust (strict)"("Visible"=w341) -> ()  [unwired: 2 in, 2 out]
        n223 = property on="Test Ring" class="Ring (strict)"("Visible"=w341) -> ()  [unwired: 2 in, 2 out]
      }
      event "Select Auto": Mouse Enter {
        # "Populate the combo box with the list of autonomous options"
        n224 = event-data() -> ()  [unwired: 1 in, 1 out]
        n225 = call <vilib>:"NT Read String Array.vi"("Name"="Auto List") -> ("String Array"=w348:string[])  [unwired: 9 in, 1 out]
        n226 = property on="Select Auto" class="CmbBox"("Strings[]"=w348) -> ()  [unwired: 2 in, 2 out]
      }
      event "Select Auto": Value Change {
        # "User modified the Auto Selection. Write to NT variable so robot knows."
        n227 = event-data() -> ("NewVal"=w351:string)  [unwired: 1 in]
        n228 = call <vilib>:"NT Write String.vi"("String"=w351, "Name"="Auto Selector") -> ()  [unwired: 9 in, 1 out]
      }
      event "Command Selection": Value Change {
        # "Get the params and show in table"
        n229 = event-data() -> ("NewVal"=w357:i32)  [unwired: 1 in]
        n230 = property on="Command Selection" class="MCListbox (strict)"() -> ("ItemNames"=w355:string[][])  [unwired: 2 in, 2 out]
        n231 = call <vilib>:"WPI_DashboardUpdate Command Params.vi"("NewVal"=w357, "Commands"=w355, "Param Tbl"=w356) -> ()  [unwired: 8 in, 1 out]
      }
      event "Execute Command": Value Change {
        # "Started one, Unique ID holds\nresponse"
        n232 = event-data() -> ()  [unwired: 1 in, 1 out]
        n233 = property on="Command Selection" class="MCListbox (strict)"() -> ("ItemNames"=w368:string[][])  [unwired: 2 in, 2 out]
        n234 = Index Array(array=w368, index (row)="Command Selection", index (col)=0) -> (element=w366:string)
        n235 = call <vilib>:"Invoke Commands.vi"("Command Params"="Command Params", "Function Name"=w366) -> ("Params"=w362:u8, "Started"=w361:bool)  [unwired: 7 in, 1 out]
        n236 = Array Subset(array="Command Params", length (row)=w362) -> (w363:string[][])  [unwired: 3 in]
        n237 = Select(t="Executing" ("Cmd Status"), s=w361, f="" ("Cmd Status")) -> (s? t:f=→"Cmd Status":string)
      }
      event "Command Selection": Double Click {
        n238 = event-data() -> ("Row"=w376:i32)  [unwired: 1 in]
        n239 = property on="Command Selection" class="MCListbox (strict)"() -> ("ItemNames"=w379:string[][])  [unwired: 2 in, 2 out]
        n240 = local read "Command Params"() -> (w375:string[][])
        n241 = Index Array(array=w379, index (row)=w376, index (col)=0) -> (element=w377:string)
        n242 = call <vilib>:"Invoke Commands.vi"("Command Params"=w375, "Function Name"=w377) -> ("Params"=w374:u8, "Started"=w369:bool)  [unwired: 7 in, 1 out]
        n243 = Array Subset(array=w375, length (row)=w374) -> (w373:string[][])  [unwired: 3 in]
        n244 = Select(t="Executing" ("Cmd Status"), s=w369, f="" ("Cmd Status")) -> (s? t:f=w370:string)
        n245 = local write "Cmd Status"(w370) -> ()
      }
      event "CheckList": Double Click {
        # "Shift clears all"
        # "Update symbols on the listbox"
        n246 = event-data() -> ("PlatMods.Shift"=w381:bool, "Row"=w383:i32)  [unwired: 1 in]
        n247 = case shown="True" w381 {
          tunnel: w383 -> [w387 _]
          tunnel: 1 -> [w386 _]
          frame False {
            n248 = property on="CheckList" class="LstBox (strict)"() -> ("Item Symbols"=w385:i32[])  [unwired: 2 in, 2 out]
            n249 = Replace Array Subset(array=w385, new element=w386, index=w387) -> (w384:i32[])
            n250 = property on="CheckList" class="LstBox (strict)"("Item Symbols"=w384) -> ()  [unwired: 2 in, 2 out]
          }
          frame True {
            w388 = 0 ("Top Row")
            n251 = property on="CheckList" class="LstBox (strict)"() -> ("Number of Rows"=w390:u32)  [unwired: 2 in, 2 out]
            n252 = Initialize Array(0, w390) -> (w389:i32[])
            n253 = property on="CheckList" class="LstBox (strict)"("Top Row"=w388, "Value"=w388, "Item Symbols"=w389) -> ()  [unwired: 2 in, 2 out]
          }
        }
      }
      event "CheckList": Key Down {
        # "Update symbols on the listbox\nLeft and right keys check and uncheck"
        n254 = event-data() -> ("VKey"=w394:T19)  [unwired: 1 in]
        n255 = case shown="\"Left\", \"Right\"" w394 {
          selector: w394 -> [w399 _]
          tunnel: eventvkey."Left" ("VKey") -> [w397 _]
          frame "Left", "Right" {
            n256 = Equal?(x=w397, y=w399) -> (x = y?=w398:bool)
            n257 = Select(t=0, s=w398, f=1) -> (s? t:f=w400:i32)
            n258 = property on="CheckList" class="LstBox (strict)"() -> ("Item Symbols"=w403:i32[])  [unwired: 2 in, 2 out]
            n259 = Replace Array Subset(array=w403, new element=w400, index="CheckList") -> (w402:i32[])
            n260 = property on="CheckList" class="LstBox (strict)"("Item Symbols"=w402) -> ()  [unwired: 2 in, 2 out]
          }
          frame Default {
          }
        }
      }
      event "Motor.Enable": Value Change {
        # "When the test mode otor enable helper is set, update that\ntree row item's value"
        n261 = event-data() -> ("NewVal"=w409:bool)  [unwired: 1 in]
        n262 = Unbundle("Motor") -> ("Value"=w408:dbl)  [unwired: 1 out]
        n263 = Select(t=w408, s=w409, f=0.0) -> (s? t:f=w406:dbl)
        n264 = call <vilib>:"NT Write Number.vi"("Numeric"=w406, "Name"=w405) -> ()  [unwired: 9 in, 1 out]
      }
      event "Test Slider": Value Change {
        # "When the test mode slider helper is set, update that\ntree row item's value"
        n265 = event-data() -> ("NewVal"=w412:dbl)  [unwired: 1 in]
        n266 = call <vilib>:"NT Write Number.vi"("Numeric"=w412, "Name"=w413) -> ()  [unwired: 9 in, 1 out]
      }
      event "On/Off": Value Change {
        # "When the test mode on/off helper value is set, update that\ntree row item's value"
        n267 = event-data() -> ("NewVal"=w417:bool)  [unwired: 1 in]
        n268 = Boolean To (0,1)(Boolean=w417) -> (0, 1=w416:i16)
        n269 = call <vilib>:"NT Write Number.vi"("Numeric"=w416, "Name"=w415) -> ()  [unwired: 9 in, 1 out]
      }
      event "Rev/Fwd": Value Change {
        # "When the test mode helper value for relays is set, update that\ntree row item's value"
        n270 = event-data() -> ("NewVal.Forward"=w425:bool, "NewVal.Reverse"=w424:bool)  [unwired: 1 in]
        n271 = Boolean To (0,1)(Boolean=w425) -> (0, 1=w421:i16)
        n272 = Boolean To (0,1)(Boolean=w424) -> (0, 1=w423:i16)
        n273 = Negate(x=w423) -> (-x=w422:i16)
        n274 = Add(x=w421, y=w422) -> (x+y=w420:i16)
        n275 = call <vilib>:"NT Write Number.vi"("Numeric"=w420, "Name"=w419) -> ()  [unwired: 9 in, 1 out]
      }
      event "Test Ring": Value Change {
        # "When a test mode helper value is selected from the ring,\nset the tree item's variable to the string value"
        n276 = event-data() -> ("NewVal"=w429:u16)  [unwired: 1 in]
        n277 = property on="Test Ring" class="Ring (strict)"() -> ("Strings []"=w430:string[])  [unwired: 2 in, 2 out]
        n278 = Index Array(array=w430, index=w429) -> (element=w428:string)
        n279 = call <vilib>:"NT Write String.vi"("String"=w428, "Name"=w427) -> ()  [unwired: 9 in, 1 out]
      }
      event "Rec Mode": Value Change {
        # "Update globals for recording mode and path to read log from.\nClear when logging and let NetworkTables set path for vision to\nuse."
        n280 = event-data() -> ("NewVal"=w441:enum32{"Stop", "Record", "Playback"})  [unwired: 1 in]
        n281 = global write "WPI_DashboardLogging Global.vi" "Logging Filename"(path "") -> ()
        n282 = global write "WPI_DashboardLogging Global.vi" "Recording"(w441) -> ()
        n283 = case shown="\"Playback\"" w441 {
          tunnel: w440 -> [_ w443 w452]
          tunnel: [_ _ w451] -> w438
          tunnel: [_ _ w450] -> _
          tunnel: w436 -> [_ _ w448]
          tunnel: cluster{i32, i32} {-250, 170} -> [_ _ w447]
          tunnel: [_ _ T20 {"Image Size"=TRUE, "Image Type"=TRUE, "Pixel Value"=TRUE, "ROI Information"=TRUE, "Zoom Factor"=FALSE} ("Image Information Shown:All Elements")] -> w434
          tunnel: [_ _ TRUE ("Zoom Factor")] -> w433
          tunnel: w432 -> [_ _ w444]
          frame Default {
          }
          frame "Stop", "Record" {
            # "Place Window too"
            n284 = invoke class="VI" method="FP.Close"(reference=w443) -> (reference out=w442:refnum<vi>)  [unwired: 2 in, 2 out]
            n285 = invoke class="VI" method="Abort VI"(reference=w442) -> ()  [unwired: 2 in, 3 out]
          }
          frame "Playback" {
            n286 = call "Open Playback Panel.vi"("Offset"=w447, "DB VI Ref"=w448, "Playback in"=w452) -> ("Playback out"=w449:refnum<vi>)  [unwired: 8 in]
            n287 = register-events(w449, w444) -> (reference out=w451:refnum<event-registration>, error out=w450:errorcluster)  [unwired: 2 in]
          }
        }
        n288 = property on="Camera Image" class="ImageControl"("Image Information Shown"=w434, "Image Information Visible"=w433) -> ()  [unwired: 2 in, 2 out]
        n289 = call <vilib>:"WPI_DashboardNT Log FieldName Cache.vi"("Operation"=enum16{"Lookup/Add", "Index", "Clear"}."Clear") -> ()  [unwired: 8 in, 3 out]
      }
      event Panel Close {
        w454 = enum32{"Stop", "Record", "Playback"}."Stop" ("Rec Mode")
        # "Playback window has been closed, abort"
        n290 = event-data() -> ()  [unwired: 1 in, 4 out]
        n291 = local write "Rec Mode"(w454) -> ()
        n292 = global write "WPI_DashboardLogging Global.vi" "Recording"(w454) -> ()
      }
      event Panel Close {
        # "Abort playback window and ourself"
        n293 = event-data() -> ()  [unwired: 1 in, 4 out]
        n294 = invoke class="VI" method="FP.Close"(reference=w458) -> (reference out=w457:refnum<vi>)  [unwired: 2 in, 2 out]
        n295 = invoke class="VI" method="Abort VI"(reference=w457) -> (error out=w456:errorcluster)  [unwired: 2 in, 2 out]
        n296 = invoke class="VI" method="Abort VI"(error in=w456) -> ()  [unwired: 2 in, 3 out]
      }
      event User Event {
        n297 = event-data() -> ("IDs"=w465:cluster{"RPC field ID":u16, "Unique ID":u16}, "String"=w464:string)  [unwired: 1 in]
        n298 = Bundle("IDs"=w465, "String"=w464) -> (w463:T8)  [unwired: 1 in]
        n299 = call <vilib>:"Retrieve RPC Response.vi"("RPC Response"=w463) -> ("Output"=w461:string[][])  [unwired: 10 in]
        n300 = Build Array (concatenate)(w459, w461) -> (w460:string[][])
        n301 = local write "Command Params"(w460) -> ()
        n302 = local write "Cmd Status"("" ("Cmd Status")) -> ()
      }
      event "Tree": Double Click {
        n303 = event-data() -> ("PlatMods"=w469:T23, "Tag"=w468:string)  [unwired: 1 in]
        n304 = Unbundle(w469) -> ("Shift"=w467:bool)  [unwired: 4 out]
        n305 = Not(x=w467) -> (.not. x?=w466:bool)
        n306 = call <vilib>:"NT Update Persistence.vi"("Persistence"=w466, "Name"=w468) -> ()  [unwired: 9 in, 1 out]
      }
    }
  }
  n307 = while {
    tunnel: w64 -> [w472]
    i -> [w475]
    stop <- FALSE stop-if-true
    n308 = Wait (ms)(milliseconds to wait=u32 100) -> ()  [unwired: 1 out]
    n309 = case shown="\"Playback\"" "Rec Mode" {
      tunnel: w475 -> [_ _ w490]
      tunnel: [u32 2829099 ("Base Color") u32 11141120 ("Target Color") w479] -> w471
      frame "Stop", Default {
        # "Reset the color, extra updates don't cost much"
      }
      frame "Record" {
      }
      frame "Playback" {
        # "Playback"
        n310 = Quotient & Remainder(x=w490, y=u32 50 ("milliseconds to wait")) -> (x-y*floor(x/y)=w486:u32)  [unwired: 1 out]
        n311 = Divide(x=w486, y=u32 50 ("milliseconds to wait")) -> (x/y=w483:dbl)
        n312 = Multiply(x=6.283185307179586, y=w483) -> (x*y=w488:dbl)
        n313 = Sine(x=w488) -> (sin(x)=w487:dbl)
        n314 = Absolute Value(x=w487) -> (abs(x)=w480:dbl)
        n315 = call "Interpolate RGB Color.vi"("Proportion"=w480, "Target Color"=u32 30976, "Base Color"=u32 2829099) -> ("Result Color"=w479:u32)  [unwired: 8 in]
      }
    }
    n316 = property class="Pane"(reference=w472, "PaneColor"=w471) -> ()  [unwired: 1 in, 2 out]
  }
  n317 = local write "Dashboard Tab"(T2."Drive" ("Dashboard Tab")) -> ()
  n318 = property on="On/Off" class="Bool (strict)"("Visible"=w33) -> ()  [unwired: 2 in, 2 out]
  n319 = property on="Motor" class="Clust (strict)"("Visible"=w33) -> ()  [unwired: 2 in, 2 out]
  n320 = property on="Progress" class="Clust (strict)"("Visible"=w33) -> ()  [unwired: 2 in, 2 out]
  n321 = property on="Test Ring" class="Ring (strict)"("Visible"=w33) -> ()  [unwired: 2 in, 2 out]
  n322 = property on="Rev/Fwd" class="Clust (strict)"("Visible"=w33) -> ()  [unwired: 2 in, 2 out]
  n323 = while {
    tunnel: u16 1741 ("timeout ms (25000)") -> [w492]
    stop <- FALSE stop-if-true
    n324 = TCP Create Listener(10:w492) -> (0:w491:errorcluster, 3:w493:refnum<k5>)  [unwired: 4 in, 1 out]
    n325 = case shown="No Error" w491 {
      selector: w491 -> [w495 _]
      tunnel: w493 -> [w496 _]
      frame No Error {
        n326 = while {
          tunnel: w496 -> [w499]
          tunnel: w495 -> [w498]
          stop <- FALSE stop-if-true
          n327 = TCP Wait On Listener(8:w498, 11:w499) -> (0:w500:errorcluster, 4:w501:refnum<k5>)  [unwired: 2 in, 3 out]
          n328 = local write "TCP"(w501) -> ()
          n329 = case shown="No Error" w500 {
            frame No Error {
            }
            frame Error {
              n330 = Wait (ms)(milliseconds to wait=u32 1000) -> ()  [unwired: 1 out]
            }
          }
        }
      }
      frame Error {
        n331 = Wait (ms)(milliseconds to wait=u32 1000) -> ()  [unwired: 1 out]
      }
    }
  }
  n332 = local write "Command Selection"(u16 0 ("milliseconds to wait")) -> ()
  n333 = local write "Command Params"(string[][] [] ("Command Params")) -> ()
  n334 = global write "WPI_DashboardLogging Global.vi" "Recording"(w58) -> ()
  n335 = local write "Rec Mode"(w58) -> ()
  n336 = call <vilib>:"NT Write String.vi"("String"="Select Auto", "Name"="Auto Selector") -> ()  [unwired: 9 in, 1 out]
